vi "global 3.vi"() -> ()   [LabVIEW 2015]
panel:
  out "배열":u8[](array[numeric])
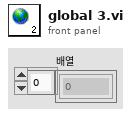
[diagram p1: front panel]
diagram:
